vi "GetType.vi"(8 "error in (no error)":errorcluster, 11 "Configure Output Mode Msg":refnum<class "Configure Output Mode Msg.lvclass">) -> (0 "error out":errorcluster, 2 "Data Sample":variant, 3 "Configure Output Mode Msg":refnum<class "Configure Output Mode Msg.lvclass">)   [LabVIEW 2016, in "CS++Fgen.lvlib" / "Configure Output Mode Msg.lvclass"]
doc: "This VI delivers a sample of the data type format the message expects."
uses:
  Configure Output Mode Msg.lvclass
  Configure Output Mode Msg.lvclass/Configure Output Mode Msg.ctl
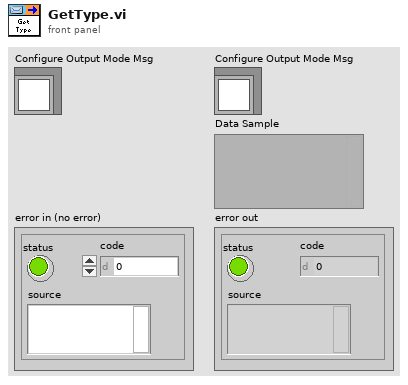
[diagram p1: front panel]
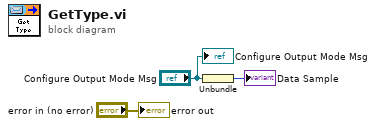
[diagram p0: block diagram]
diagram:
  n1 = Unbundle("Configure Output Mode Msg") -> (→"Data Sample":i32)
  "error out" <- "error in (no error)"
  "Configure Output Mode Msg" <- "Configure Output Mode Msg"
